vi "VIA Minify VI Locals.vi"(11 "VIA in":string) -> (1 "Bytes Removes":i32, 2 "Num Locals - 1":i32, 3 "VIA out":string)   [LabVIEW 2020]
uses:
  <vilib>/regexp/Match Regular Expression.xnode
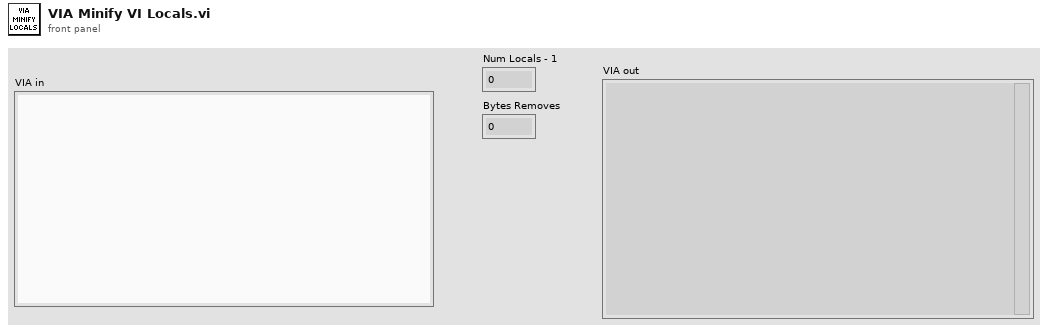
[diagram p1: front panel]
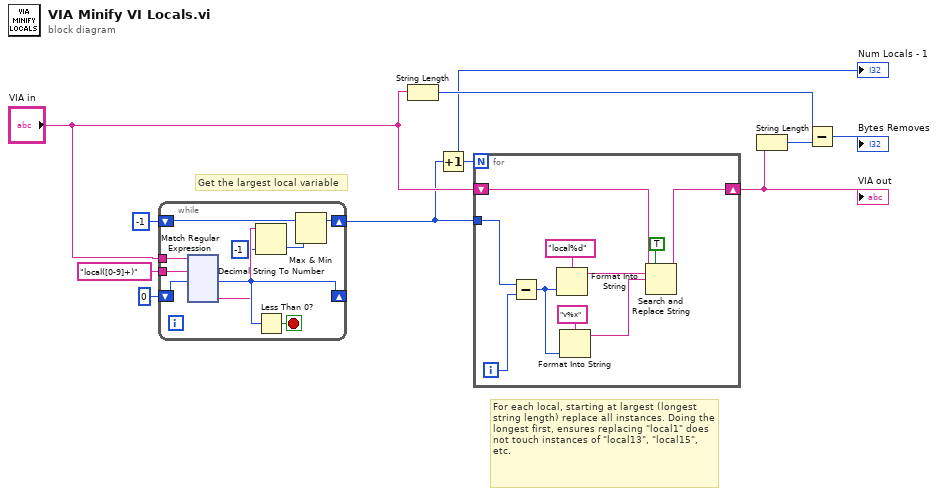
[diagram p0: block diagram]
diagram:
  # "For each local, starting at largest (longest string length) replace all instances. Doing the longest first, ensures replacing \"local1\" does not touch instances of \"local13\", \"local15\", etc."
  # "Get the largest local variable"
  n1 = while {
    tunnel: "local([0-9]+)" ("regular expression") -> [w20]
    shift-right: [w16] -> _
    shift-left: 0 ("offset past match") -> [w18]
    shift-right: [w12] -> w2
    shift-left: -1 -> [w14]
    tunnel: "VIA in" -> [w19]
    stop <- w17 stop-if-true
    n2 = xnode "Match Regular Expression"("input string"=w19, "regular expression"=w20, "offset (0)"=w18) -> ("offset past match"=w16:i32, "submatch 1"=w15:string)  [unwired: 3 in, 4 out]
    n3 = Decimal String To Number(string=w15, default (0L)=-1 ("default (0 I32)")) -> (number=w13:i32)  [unwired: 1 in, 1 out]
    n4 = Less Than 0?(x=w16) -> (x < 0?=w17:bool)
    n5 = Max & Min(x=w14, y=w13) -> (max(x,y)=w12:i32)  [unwired: 1 out]
  }
  n6 = String Length(string="VIA in") -> (length=w4:i32)
  n7 = Increment(x=w2) -> (x+1=w1:i32)
  "Num Locals - 1" <- w1
  n8 = for {
    N: w1 -> [_]
    tunnel: w2 -> [w146]
    shift-right: [w137] -> w6
    shift-left: "VIA in" -> [w143]
    i -> [w145]
    n9 = Subtract(x=w146, y=w145) -> (x-y=w140:i32)
    n10 = Format Into String(format string="local%d", w140) -> (resulting string=w142:string)  [unwired: 2 in, 1 out]
    n11 = Format Into String(format string="v%x", w140) -> (resulting string=w139:string)  [unwired: 2 in, 1 out]
    n12 = Search and Replace String(replace all?=TRUE ("replace all? (F)"), input string=w143, search string=w142, replace string=w139) -> (result string=w137:string)  [unwired: 4 in, 3 out]
  }
  "VIA out" <- w6
  n13 = String Length(string=w6) -> (length=w5:i32)
  n14 = Subtract(x=w4, y=w5) -> (x-y=→"Bytes Removes":i32)
